vi "parse file data.vi"(8 "error in":errorcluster, 11 "file format":T6) -> (0 "error out":errorcluster, 3 "file information":T1)   [LabVIEW 2013, in "PLConfigurationSerializer.lvlib"]
uses:
  PLConfigurationSerializer.lvlib
  file format.ctl
  1_0_0_0 format.ctl
  system hierarchy.ctl
  target hierarchy.ctl
  engine hierarchy.ctl
  configuration database.ctl
  <vilib>/NI/Configuration Framework/serializable configuration/NISE_CEF_serializable configuration.lvclass
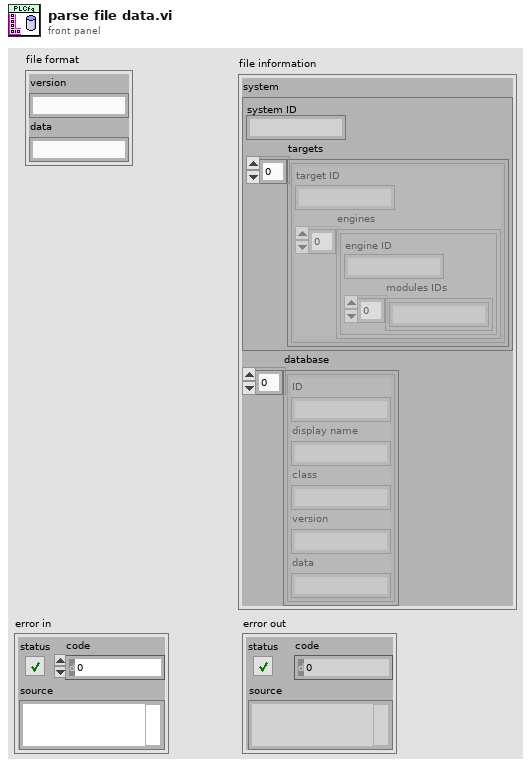
[diagram p1: front panel]
types:
  T1 = typedef "PLConfigurationSerializer.lvlib/1_0_0_0 format.ctl" = cluster{"system":T2, "database":T5[]}
  T2 = typedef "PLConfigurationSerializer.lvlib/system hierarchy.ctl" = cluster{"system ID":string, "targets":T3[]}
  T3 = typedef "PLConfigurationSerializer.lvlib/target hierarchy.ctl" = cluster{"target ID":string, "engines":T4[]}
  T4 = typedef "PLConfigurationSerializer.lvlib/engine hierarchy.ctl" = cluster{"engine ID":string, "modules IDs":string[]}
  T5 = typedef "PLConfigurationSerializer.lvlib/configuration database.ctl" = cluster{"ID":string, "display name":string, "class":string, "version":string, "data":string}
  T6 = typedef "PLConfigurationSerializer.lvlib/file format.ctl" = cluster{"version":string, "data":string}
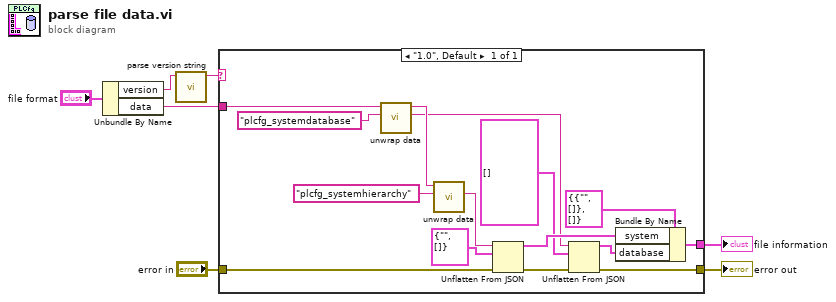
[diagram p0: block diagram]
diagram:
  n1 = Unbundle By Name("file format") -> ("version"=w6:string, "data"=w2:string)
  n2 = call <vilib>:"parse version string.vi"("full version"=w6) -> ("major.minor version"=w5:string)  [unwired: 7 in, 3 out]
  n3 = case shown="\"1.0\", Default" w5 {
    tunnel: "error in" -> [w22]
    tunnel: [w11] -> w3
    tunnel: w2 -> [w18]
    tunnel: [w19] -> w1
    frame "1.0", Default {
      n4 = call <vilib>:"unwrap data.vi"("identifier"="plcfg_systemdatabase", "data to unwrap"=w18) -> ("unwrapped data"=w9:string, "remaining string"=w17:string)  [unwired: 8 in]
      n5 = call <vilib>:"unwrap data.vi"("identifier"="plcfg_systemhierarchy", "data to unwrap"=w17) -> ("unwrapped data"=w13:string)  [unwired: 8 in, 1 out]
      n6 = Unflatten From JSON(JSON string=w13, type and defaults=T2 {"system ID"="", "targets"=[]} ("system"), error in (no error)=w22) -> (value=w12:T2, error out=w21:errorcluster)  [unwired: 4 in]
      n7 = Unflatten From JSON(JSON string=w9, type and defaults=T5[] [] ("database"), error in (no error)=w21) -> (value=w8:T5[], error out=w11:errorcluster)  [unwired: 4 in]
      n8 = Bundle By Name(cluster=T1 {"system"={"system ID"="", "targets"=[]}, "database"=[]} ("file information"), "system"=w12, "database"=w8) -> (w19:T1)
    }
  }
  "error out" <- w3
  "file information" <- w1
